vi "rearrange_points.vi"(8 "error in (no error)":errorcluster, 11 "TrajectoryDL121017Hopping in":refnum<class "TrajectoryDL121017Hopping.lvclass">) -> (0 "error out":errorcluster, 3 "TrajectoryDL121017Hopping out":refnum<class "TrajectoryDL121017Hopping.lvclass">)   [LabVIEW 2010, in "TrajectoryDL121017Hopping.lvclass"]
doc: "Rearranges clockwise sorted points to further reduce path length. See PhD thesis by Werner Göbel (section 2.1.3.2) for details."
uses:
  TrajectoryDL121017Hopping.lvclass
  TrajectoryDL121017Hopping.lvclass/TrajectoryDL121017Hopping.ctl
  common/classes/SpaceVector/SpaceVector/SpaceVector.lvclass
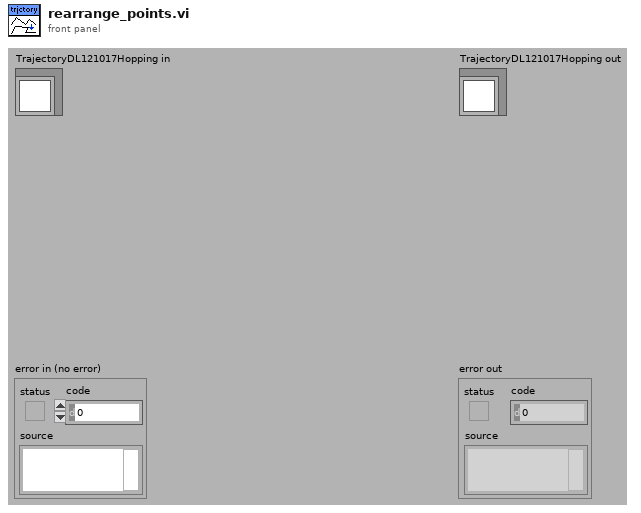
[diagram p1: front panel]
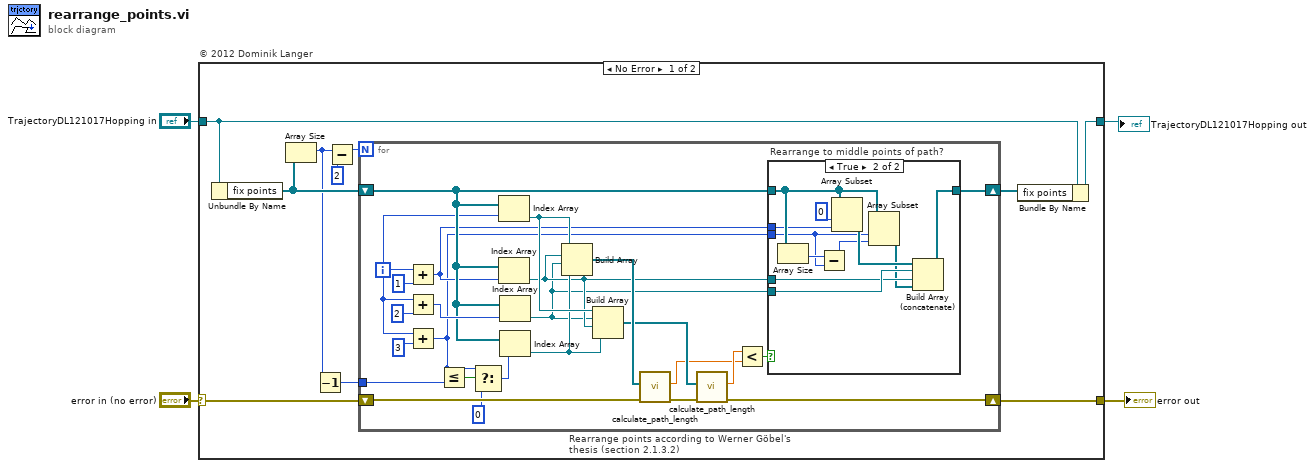
[diagram p0: block diagram]
diagram:
  n1 = case "© 2012 Dominik Langer" shown="No Error" "error in (no error)" {
    selector: "error in (no error)" -> [w14 w53]
    tunnel: [w13 w53] -> w1
    tunnel: [w10 w52] -> w2
    tunnel: "TrajectoryDL121017Hopping in" -> [w11 w52]
    frame No Error {
      n2 = Unbundle By Name(w11) -> ("fix points"=w9:refnum<class "SpaceVector.lvclass">[])
      n3 = Array Size(array=w9) -> (size(s)=w6:i32)
      n4 = Decrement(x=w6) -> (x-1=w5:i32)
      n5 = Subtract(x=w6, y=2) -> (x-y=w8:i32)
      n6 = for "Rearrange points according to Werner Göbel's thesis (section 2.1.3.2)" {
        N: w8 -> [_]
        shift-right: [w33] -> w13
        shift-left: w14 -> [w35]
        shift-right: [w24] -> w12
        shift-left: w9 -> [w25]
        tunnel: w5 -> [w19]
        i -> [w23]
        n7 = Add(x=w23, y=1) -> (x+y=w20:i32)
        n8 = Add(x=w23, y=2) -> (x+y=w36:i32)
        n9 = Add(x=w23, y=3) -> (x+y=w17:i32)
        n10 = Less Or Equal?(x=w17, y=w19) -> (x <= y?=w18:bool)
        n11 = Select(t=w17, s=w18, f=0) -> (s? t:f=w16:i32)
        n12 = Index Array(array=w25, index=w23) -> (element=w32:refnum<class "SpaceVector.lvclass">)
        n13 = Index Array(array=w25, index=w20) -> (element=w22:refnum<class "SpaceVector.lvclass">)
        n14 = Index Array(array=w25, index=w36) -> (element=w21:refnum<class "SpaceVector.lvclass">)
        n15 = Index Array(array=w25, index=w16) -> (element=w31:refnum<class "SpaceVector.lvclass">)
        n16 = Build Array(w32, w22, w21, w31) -> (w30:refnum<class "SpaceVector.lvclass">[])
        n17 = Build Array(w32, w21, w22, w31) -> (w29:refnum<class "SpaceVector.lvclass">[])
        n18 = call "calculate_path_length.vi"("error in (no error)"=w35, "path in"=w30) -> ("error out"=w34:errorcluster, "length"=w27:dbl[unit])  [unwired: 8 in]
        n19 = call "calculate_path_length.vi"("error in (no error)"=w34, "path in"=w29) -> ("error out"=w33:errorcluster, "length"=w28:dbl[unit])  [unwired: 8 in]
        n20 = Less?(x=w28, y=w27) -> (x < y?=w26:bool)
        n21 = case "Rearrange to middle points of path?" shown="True" w26 {
          tunnel: w25 -> [w40 w46]
          tunnel: [w40 w47] -> w24
          tunnel: w22 -> [_ w48]
          tunnel: w21 -> [_ w49]
          tunnel: w20 -> [_ w45]
          tunnel: w17 -> [_ w43]
          frame False {
          }
          frame True {
            n22 = Array Size(array=w46) -> (size(s)=w44:i32)
            n23 = Subtract(x=w44, y=w43) -> (x-y=w42:i32)
            n24 = Array Subset(array=w46, index=0, length=w45) -> (w50:refnum<class "SpaceVector.lvclass">[])
            n25 = Array Subset(array=w46, index=w43, length=w42) -> (w41:refnum<class "SpaceVector.lvclass">[])
            n26 = Build Array (concatenate)(w50, w49, w48, w41) -> (w47:refnum<class "SpaceVector.lvclass">[])
          }
        }
      }
      n27 = Bundle By Name(cluster=w11, "fix points"=w12) -> (w10:refnum<class "TrajectoryDL121017Hopping.lvclass">)
    }
    frame Error {
    }
  }
  "error out" <- w1
  "TrajectoryDL121017Hopping out" <- w2
